vi "Find And Load Measurement.vi"(8 "error in (no error)":errorcluster, 9 "Reset Defaults":bool=TRUE, 10 "data in":T1, 11 "Queue in":refnum<queue>) -> (0 "error out":errorcluster, 2 "data out":T1, 3 "dup Queue in":refnum<queue>)   [LabVIEW 2020, in "InstrumentStudioPlugin.lvlib"]
uses:
  InstrumentStudioPlugin.lvlib
  controls/Data.ctl
  Measurement Client Wrapper/Measurement Client Wrapper.lvclass
  Message Queue/Message Cluster.ctl
  Message Queue/Message Queue.lvlib
  Message Queue/Enqueue Message (Array).vi
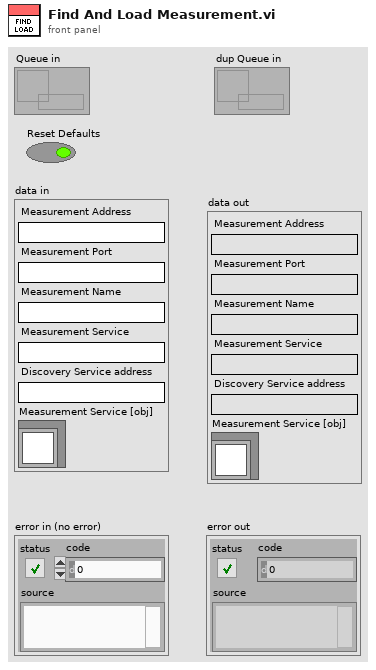
[diagram p1: front panel]
types:
  T1 = typedef "InstrumentStudioPlugin.lvlib/Data.ctl" = cluster{"Measurement Address":string, "Measurement Port":string, "Measurement Name":string, "Measurement Service":string, "Discovery Service address":string, "Measurement Service [obj]":refnum<class "Measurement Client Wrapper.lvclass">}
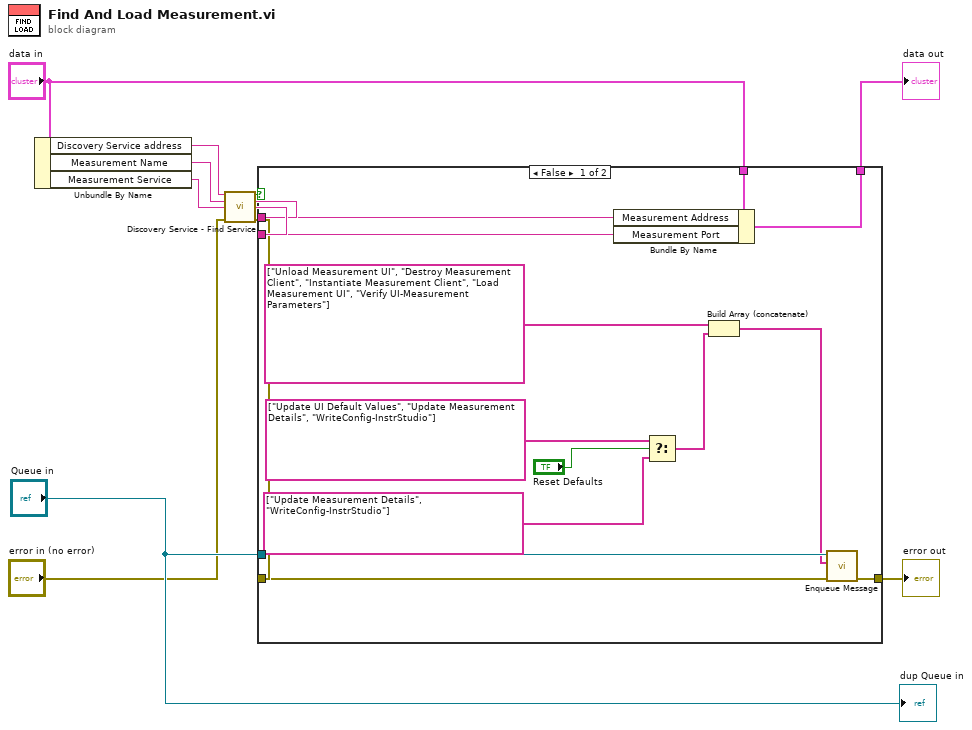
[diagram p0: block diagram]
diagram:
  n1 = Unbundle By Name("data in") -> ("Discovery Service address"=w10:string, "Measurement Name"=w11:string, "Measurement Service"=w12:string)
  n2 = call "Discovery Service - Find Service.vi"("discovery address"=w10, "Measurement Name"=w11, "Measurement Service"=w12, "error in"="error in (no error)") -> ("Cancelled?"=w2:bool, "Measurement location"=w6:string, "Measurement port"=w7:string, "error out"=w4:errorcluster)  [unwired: 8 in]
  n3 = case shown="False" w2 {
    tunnel: "Queue in" -> [w25 _]
    tunnel: w4 -> [w24 w27]
    tunnel: [w23 w27] -> w5
    tunnel: w6 -> [w21 _]
    tunnel: w7 -> [w20 _]
    tunnel: "data in" -> [w22 w26]
    tunnel: [w19 w26] -> w8
    frame False {
      n4 = Bundle By Name(cluster=w22, "Measurement Address"=w21, "Measurement Port"=w20) -> (w19:T1)
      n5 = Select(t=string[] ["Update UI Default Values", "Update Measurement Details", "WriteConfig-InstrStudio"], s="Reset Defaults", f=string[] ["Update Measurement Details", "WriteConfig-InstrStudio"]) -> (s? t:f=w18:string[])
      n6 = Build Array (concatenate)(string[] ["Unload Measurement UI", "Destroy Measurement Client", "Instantiate Measurement Client", "Load Measurement UI", "Verify UI-Measurement Parameters"], w18) -> (w13:string[])
      n7 = call-poly "Enqueue Message.vi"("error in (no error)"=w24, "Message Array"=w13, "Message Queue"=w25) -> ("error out"=w23:errorcluster)  [unwired: 7 in, 1 out]
    }
    frame True {
    }
  }
  "data out" <- w8
  "error out" <- w5
  "dup Queue in" <- "Queue in"
